vi "UI.vi"(0 "reference in":refnum<class "GUI OIL_FILLING.lvclass">, 5 "error in (no error)":errorcluster) -> (14 "reference out":refnum<class "GUI OIL_FILLING.lvclass">, 19 "error out":errorcluster)   [LabVIEW 2019, in "GUI OIL_FILLING.lvclass"]
uses:
  GUI OIL_FILLING.lvclass
  D:/H4000/src/GUI_class/GUI.lvclass
  GUI_class/GUI.lvclass/GUI.ctl
  TypeDef/AI_Data_Array.ctl
  TypeDef/AI_Data.ctl
  SV_Wrap/SharedVariableWrapper.lvclass/SharedVariableWrapper.ctl
  TypeDef/State.ctl
  MessageAMC_class/MessageAMC.lvclass
  D:/H4000/src/MessageInterface_class/MessageInterface.lvclass
  60afc6ad-d234-470a-b2ea-5a97dad0136d.vi
  94cfafae-4fb1-41fa-8c91-5db137de6dca.vi
  1b4fed76-272f-4eb9-b435-1b7916789d73.vi
  d0ca9bf2-7cd9-4c29-a03d-de1c10393a74.vi
  GUI_class/Set Win State.vi
  94cfafae-4fb1-41fa-8c91-5db137de6dca.vi/4db0cfde-7309-4fb5-ba82-78d4deda94bf.vi
  SV_Wrap/Write Var Info.vi
  SV_Wrap/Read Var Info.vi
  1b4fed76-272f-4eb9-b435-1b7916789d73.vi/fad6aa2d-1fd6-40e9-9208-cebdd25b163b.vi
  d0ca9bf2-7cd9-4c29-a03d-de1c10393a74.vi/ea186c4c-0445-4979-bfc0-5907181f2b8f.vi
  SV_Wrap/Read connection str.vi
  <userlib>/_OpenG.lib/time/time.llb/Tick Count (ms)__ogtk.vi
  TypeDef/GUI Setting Channel.ctl
  GUI_class/GUI.lvclass
  ConfigInterface_class/ConfigInterface.lvclass
  d678bd6a-011c-496f-8712-f7d087665a22.vi
  8e32a023-0563-484b-b85f-c3305c0d5712.vi
  MessageInterface_class/MessageInterface.lvclass
  SV_Wrap/SharedVariableWrapper.lvclass
panel:
  out "State":string
  in  "Set SP":bool
  in  "Setpoint":dbl caption="Давление прокачки"
  in  "Stop Button":bool
  in  "Start Button":bool
  out "AI 9":dbl(knob) caption="Давление  в  линии подачи \nвоздуха после БПВ" scale=0.0..16.0
  out "AI 8":dbl(knob) caption="Давление  в  линии подачи \nвоздуха в БПВ" scale=0.0..16.0
  out "DI 11":bool caption="БП [G2]"
  out "DI 8":bool caption="QF9"
  out "DI 7":bool caption="QF8"
  out "DI 6":bool caption="QF7"
  out "DI 5":bool caption="QF6"
  out "DI 4":bool caption="QF5"
  out "DI 3":bool caption="QF4"
  out "DI 2":bool caption="QF3"
  out "DI 1":bool caption="QF2"
  out "DI 0":bool caption="QF1"
  out "Connect":bool
  in  "Reset Alarms":bool
  in  "stop":bool
  out "DI 10":bool caption="БП [G1]"
  out "DI 9":bool caption="РКФ"
  # "Автоматы"
  # "0 - не готов\n1 -готов к запуска\n2 - пуск\n3 -качает\n4 - отскановка"
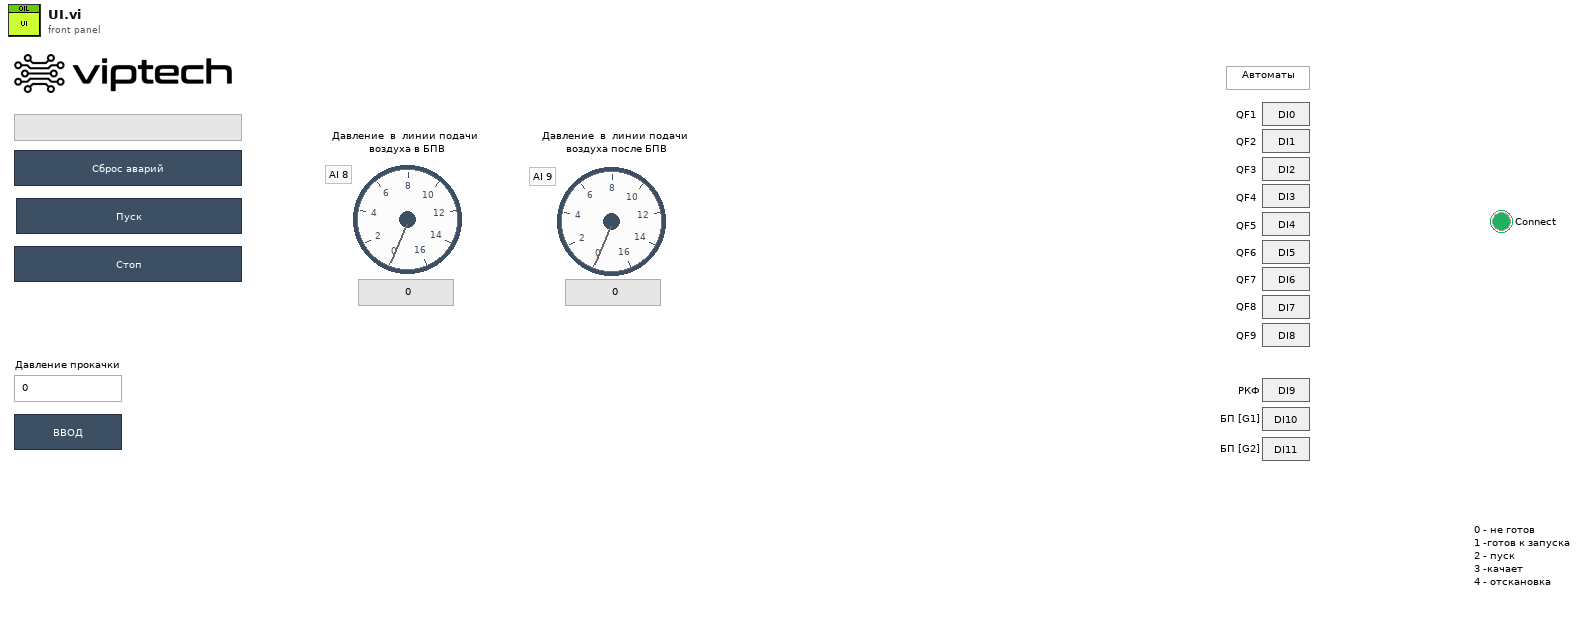
[diagram p1: front panel]
types:
  T1 = typedef "State.ctl" = enum16{"INIT", "IDLE", "CHANNEL_TESTING", "OIL_FILLING", "PREPARE_TO_HI_PRESS", "HI_PRESSURE", "ALARM", "HI PRESSURE TEST"}
  T2 = enum32{"Invalid", "Standard", "Closed", "Hidden", "Minimized", "Maximized"}
  T3 = enum32{"invalid app kind", "Development System", "Run Time System", "Student Edition", "Embedded LabVIEW", "Evaluation", "Custom"}
  T4 = typedef "GUI Setting Channel.ctl" = cluster{"Name":string, "SensorID":u32}
  T5 = typedef "GUI.lvclass/Shered Data.ctl" = cluster{"WindowsState":T6, "UI VI":refnum<vi>, "SubPnl":refnum<vi>}
  T6 = typedef "GUI.lvclass/WindowsState.ctl" = enum16{"NotReady", "Ready", "Inserted", "Opened"}
  T7 = typedef "SharedVariableWrapper.lvclass/Config.ctl" = cluster{"connection str":string, "timeout":dbl, "ip":string}
  T8 = cluster{"Core":cluster{"Current VI Reference":refnum<vi>, "Close Panel on Exit?":bool}, "amc":refnum<class "MessageAMC.lvclass">}
  T9 = cluster{"Current VI Reference":refnum<vi>, "Close Panel on Exit?":bool}
  T10 = typedef "GUI Alarm customer settings.ctl" = cluster{"HIHI AI2":dbl, "HI AI2":dbl, "HIHI AI3":dbl, "HI AI3":dbl, "ENG0 OFF TIMEOUT":dbl, "ENG0 ON TIMEOUT":dbl, "HIHI AI7":dbl, "HI AI7":dbl, "HIHI AI6":dbl, "HI AI6":dbl, "HIHI AI5":dbl, "HI AI5":dbl}
  T11 = typedef "GUI Alarm developer settings.ctl" = cluster{"HIHI AI2":dbl, "HI AI2":dbl, "HIHI AI0":dbl, "HI AI0":dbl, "LOLO AI0":dbl, "LO AI0":dbl, "ENG2 OFF TIMEOUT":dbl, "ENG2 ON TIMEOUT":dbl, "HIHI AI3":dbl, "HI AI3":dbl, "HIHI AI1":dbl, "HI AI1":dbl, "LOLO AI1":dbl, "LO AI1":dbl, "ENG1 OFF TIMEOUT":dbl, "ENG1 ON TIMEOUT":dbl, "ENG0 OFF TIMEOUT":dbl, "ENG0 ON TIMEOUT":dbl, "LOLO AI8":dbl, "LO AI8":dbl, "LOLO AI9":dbl, "LO AI9":dbl, "LOLO AI5":dbl, "LO AI5":dbl, "Out Of Range HI":dbl, "Out Of Range LO":dbl}
  T12 = typedef "AI_Data_Array.ctl" = T13[]
  T13 = typedef "AI_Data.ctl" = cluster{"Raw":dbl, "Scaled":dbl, "OutOfRangeMax":bool, "OutOfRangeMin":bool, "HIHI":bool, "HI":bool, "LO":bool, "LOLO":bool, "OutOfRangeMax_val":dbl, "OutOfRangeMin_val":dbl, "HIHI_val":dbl, "HI_val":dbl, "LO_val":dbl, "LOLO_val":dbl}
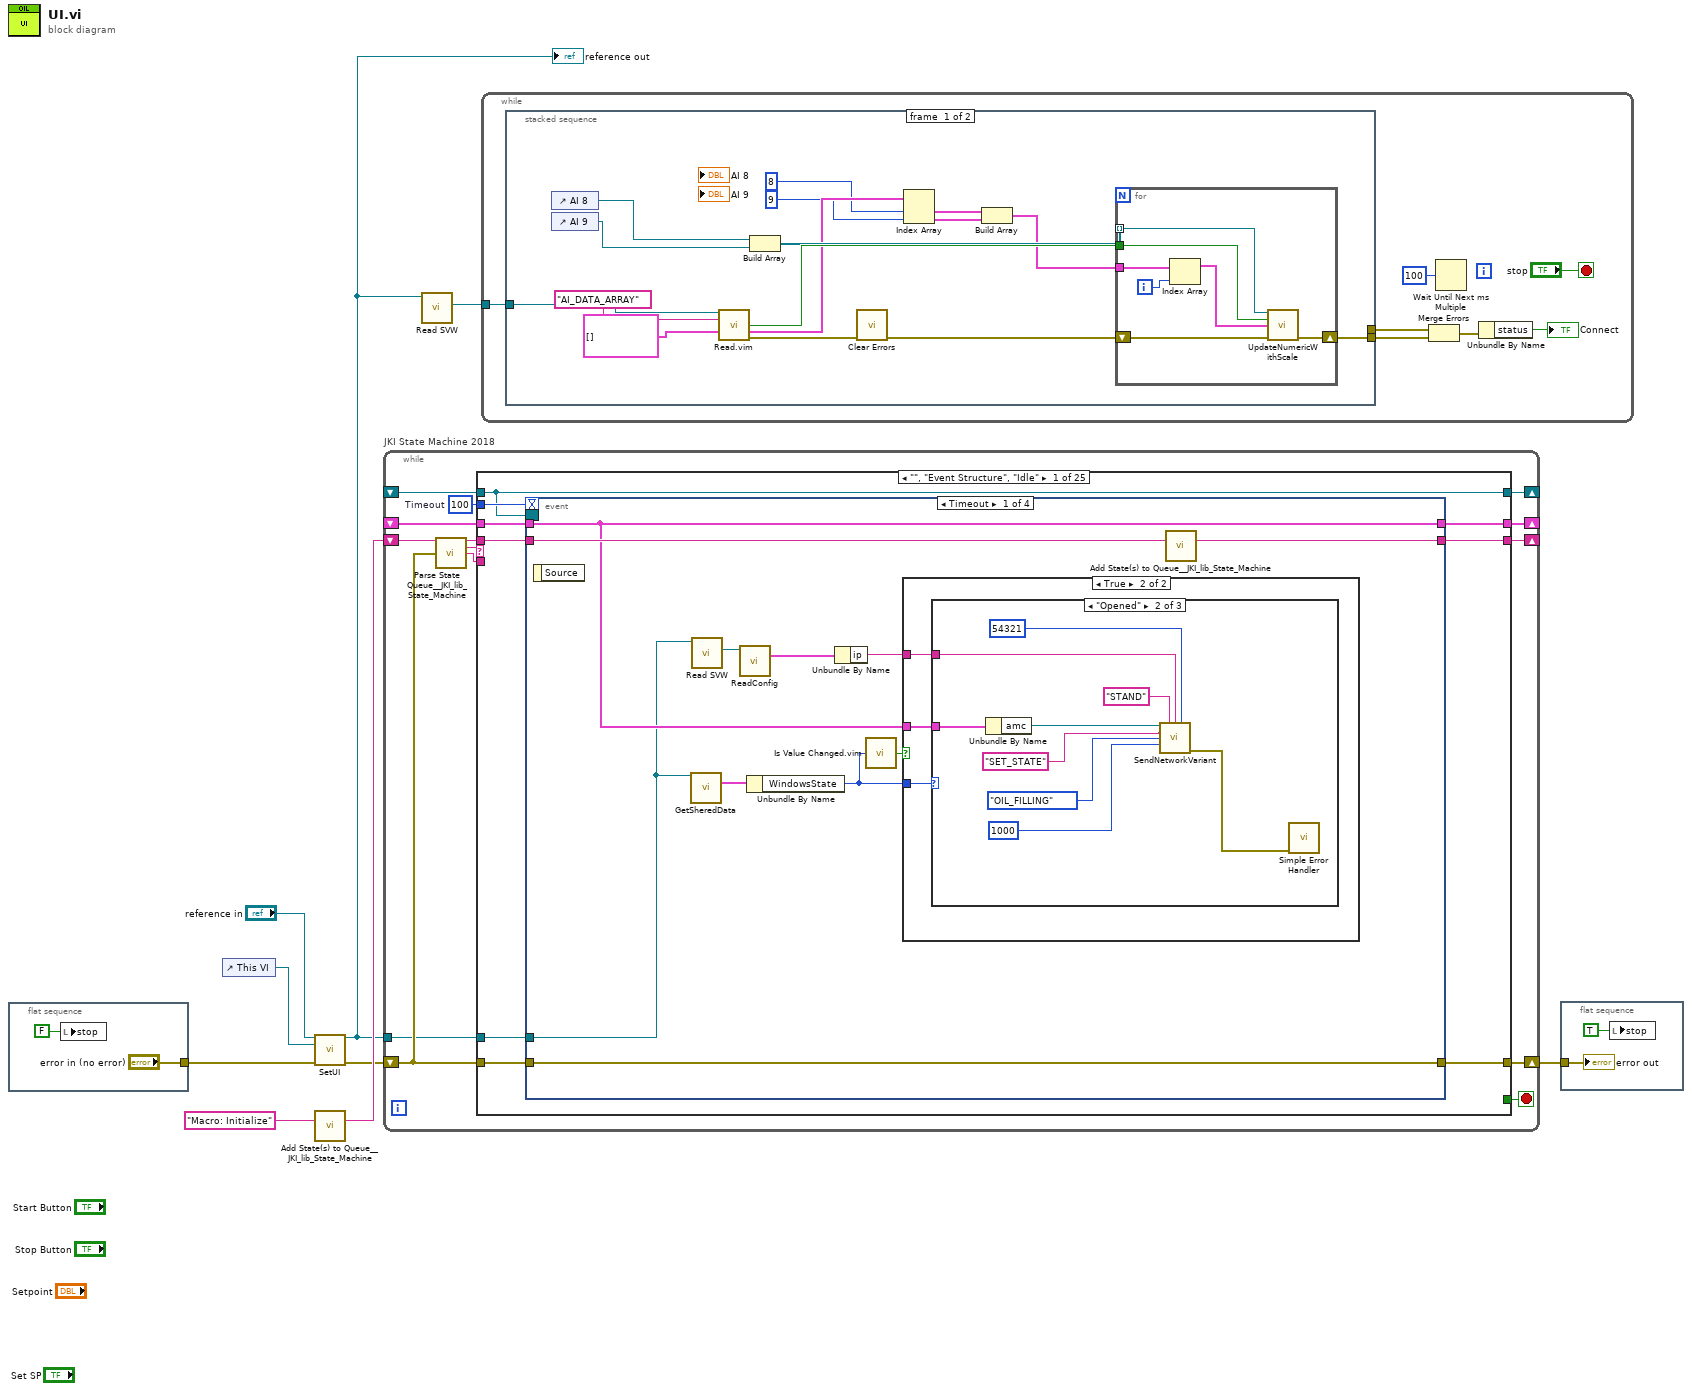
[diagram p0: block diagram]
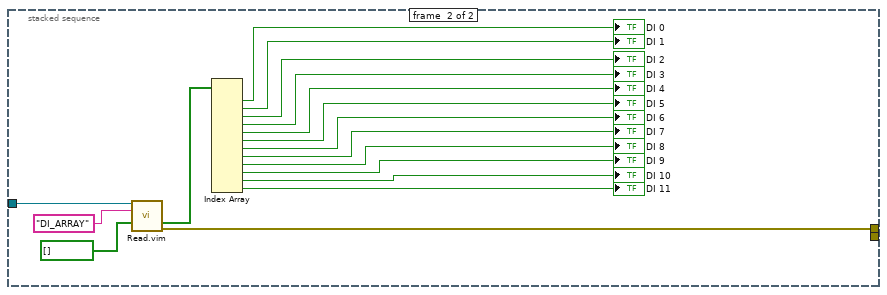
[diagram p2: hidden frame]
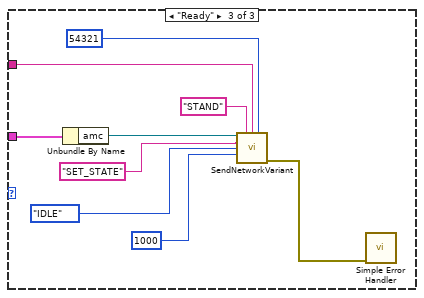
[diagram p5: hidden frame]
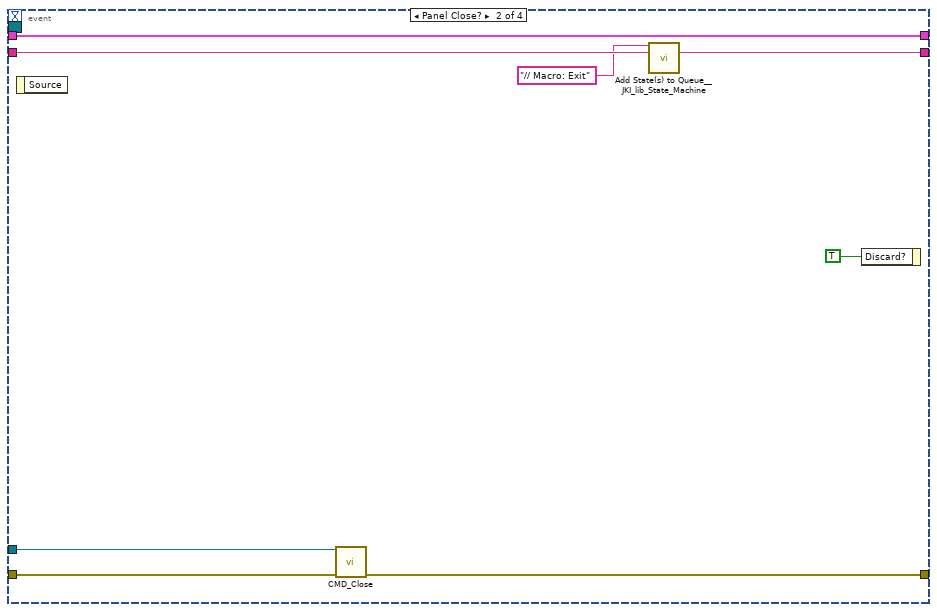
[diagram p6: hidden frame]
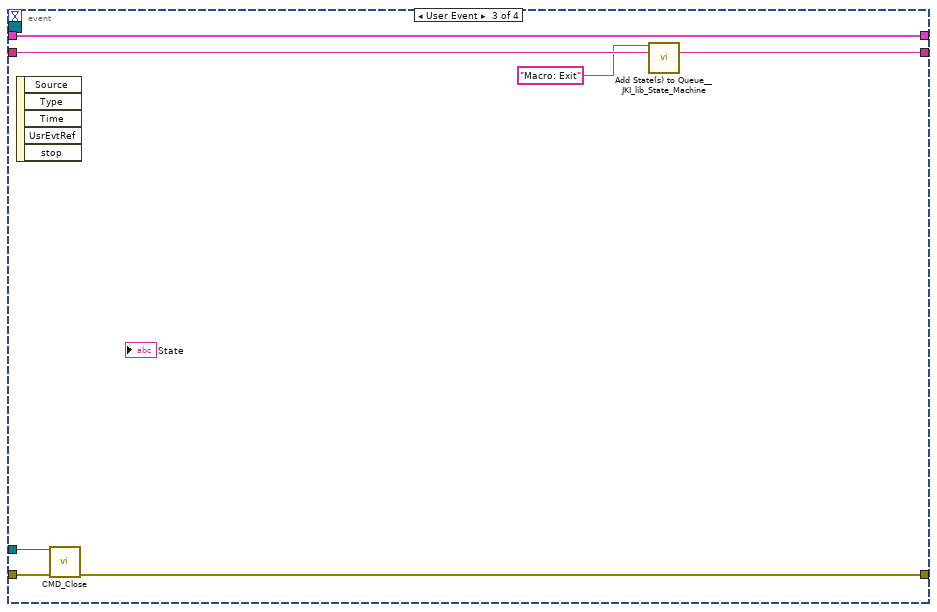
[diagram p7: hidden frame]
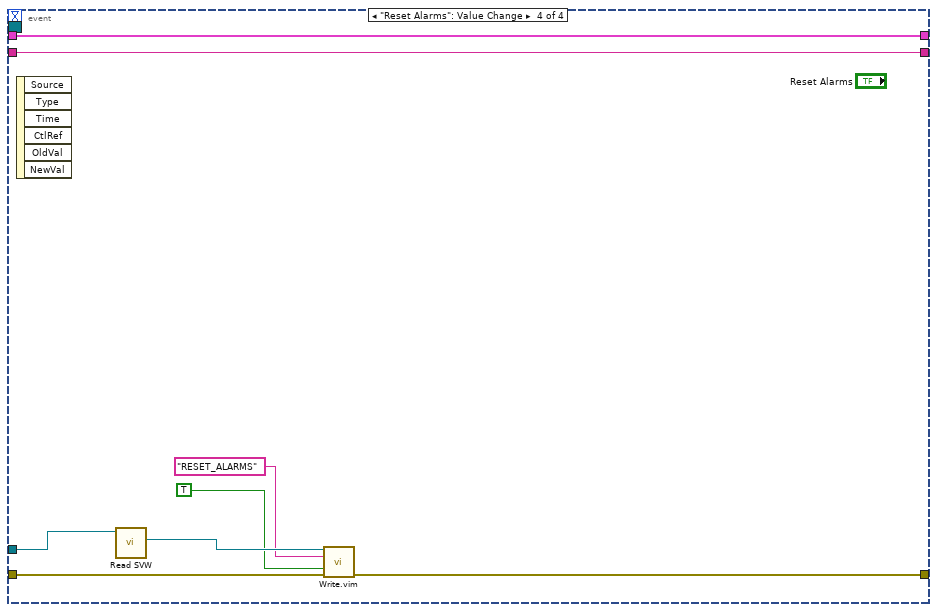
[diagram p8: hidden frame]
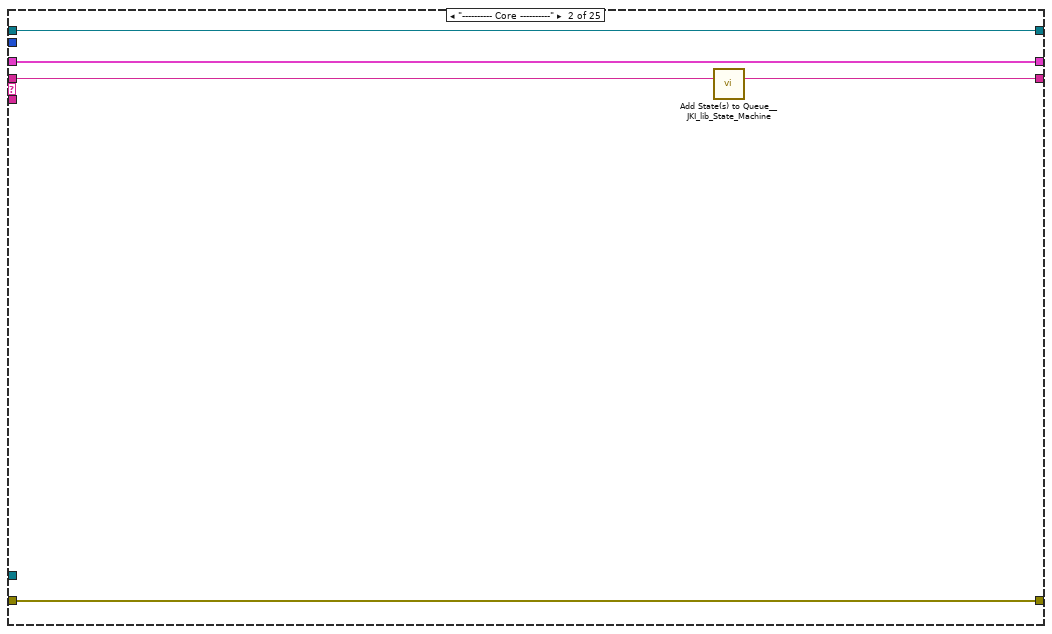
[diagram p9: hidden frame]
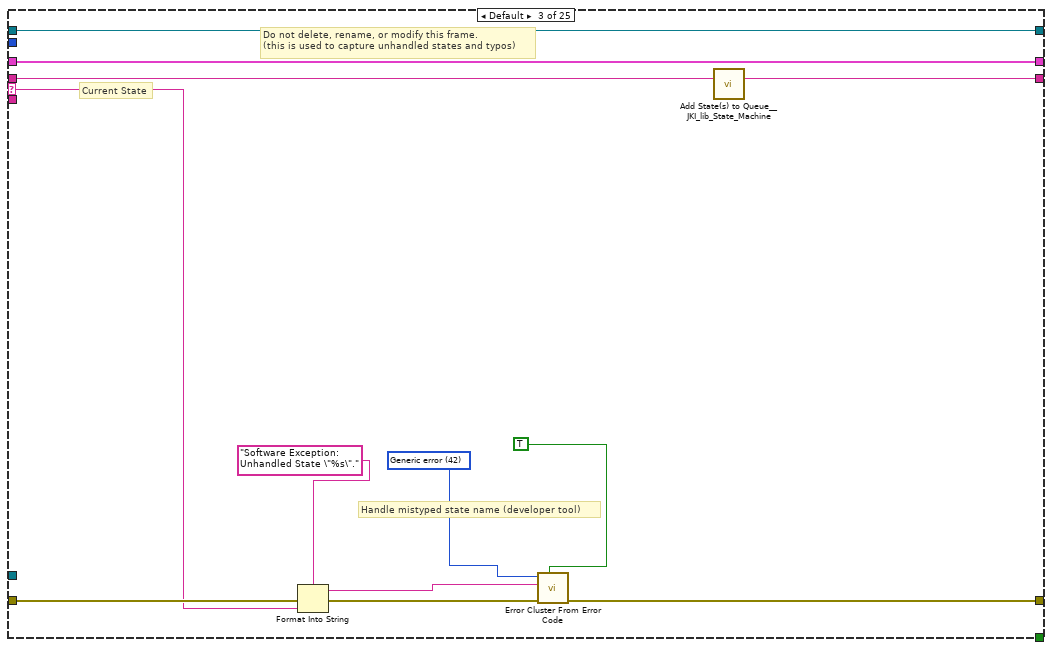
[diagram p10: hidden frame]
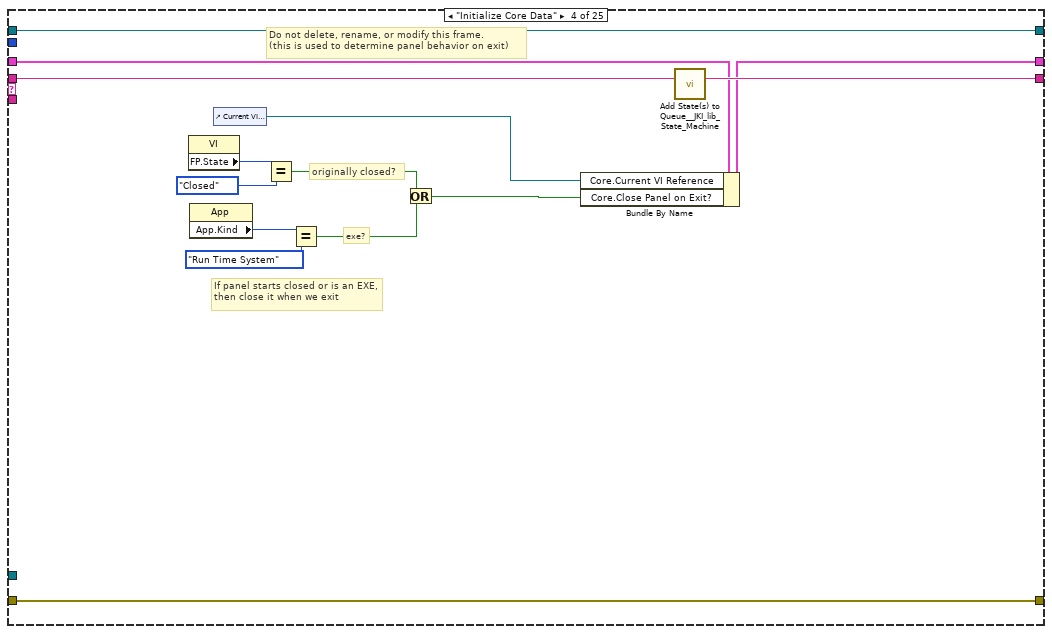
[diagram p11: hidden frame]
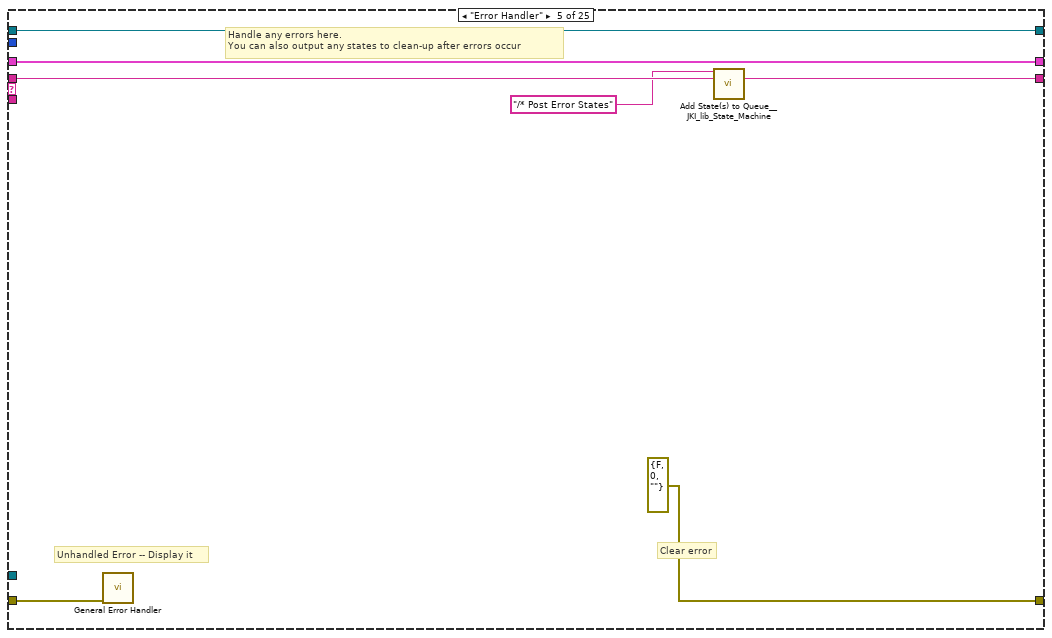
[diagram p12: hidden frame]
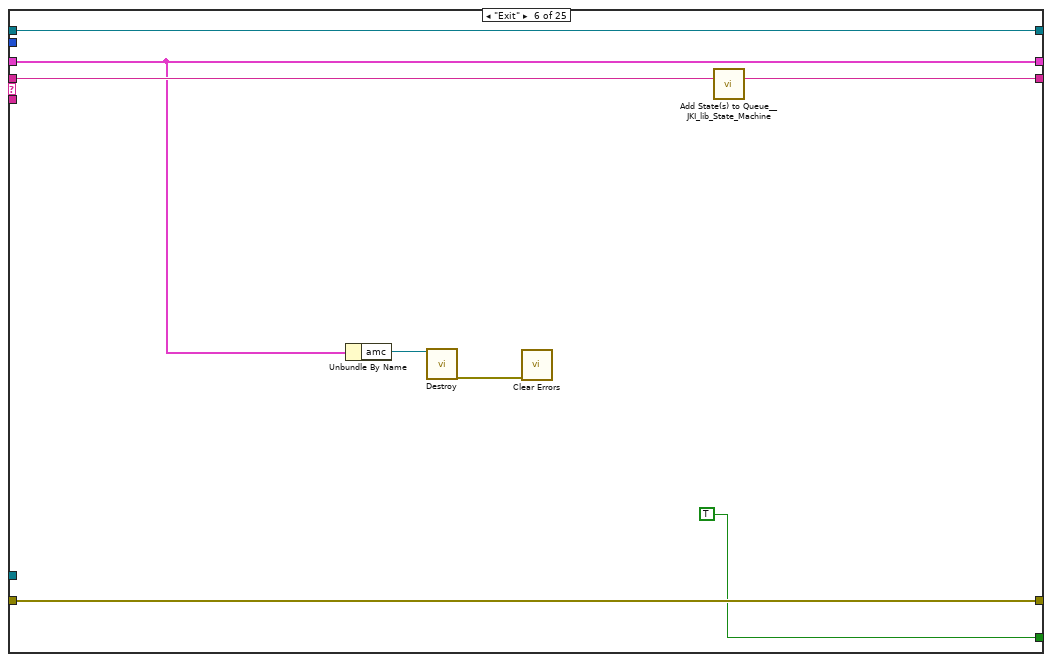
[diagram p13: hidden frame]
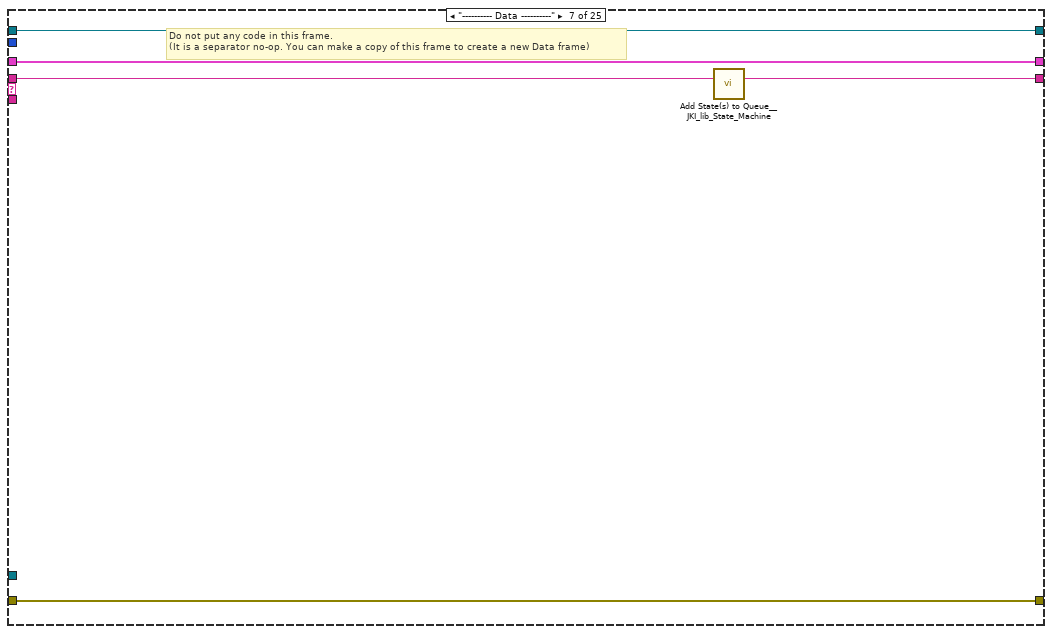
[diagram p14: hidden frame]
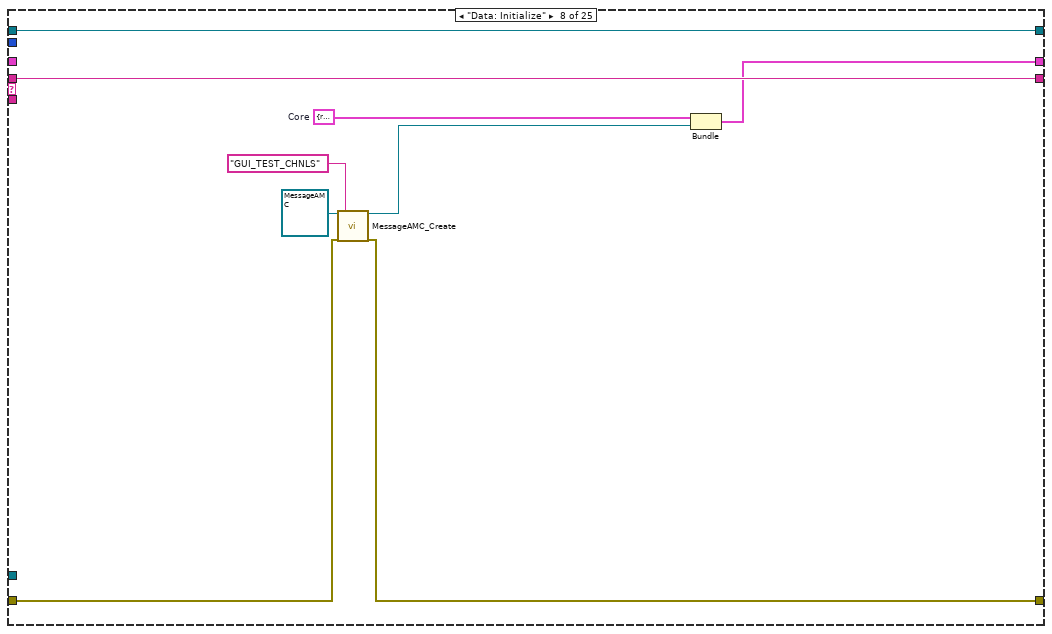
[diagram p15: hidden frame]
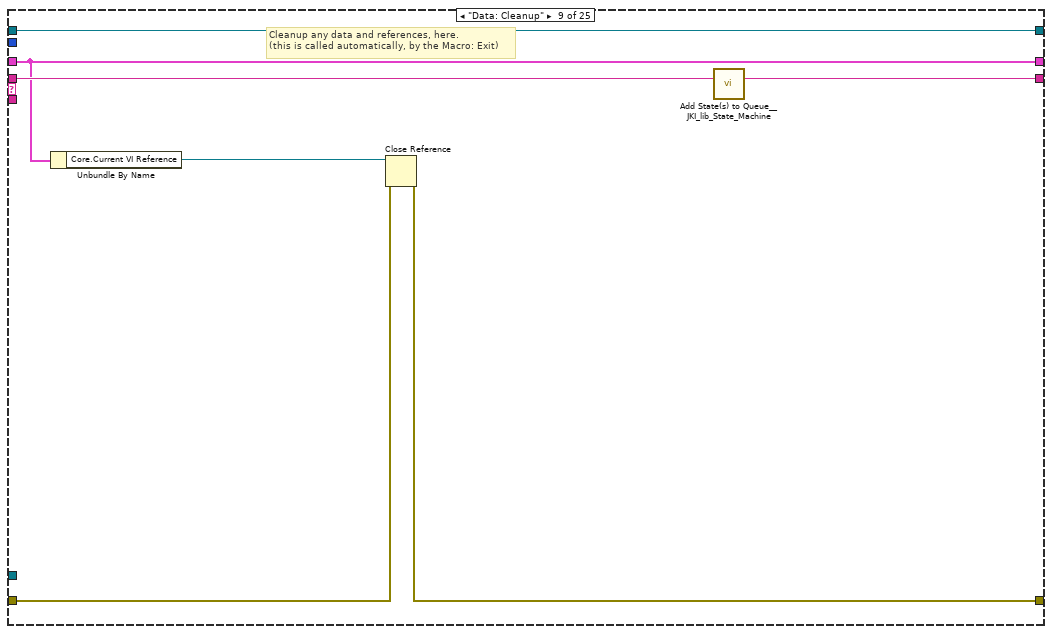
[diagram p16: hidden frame]
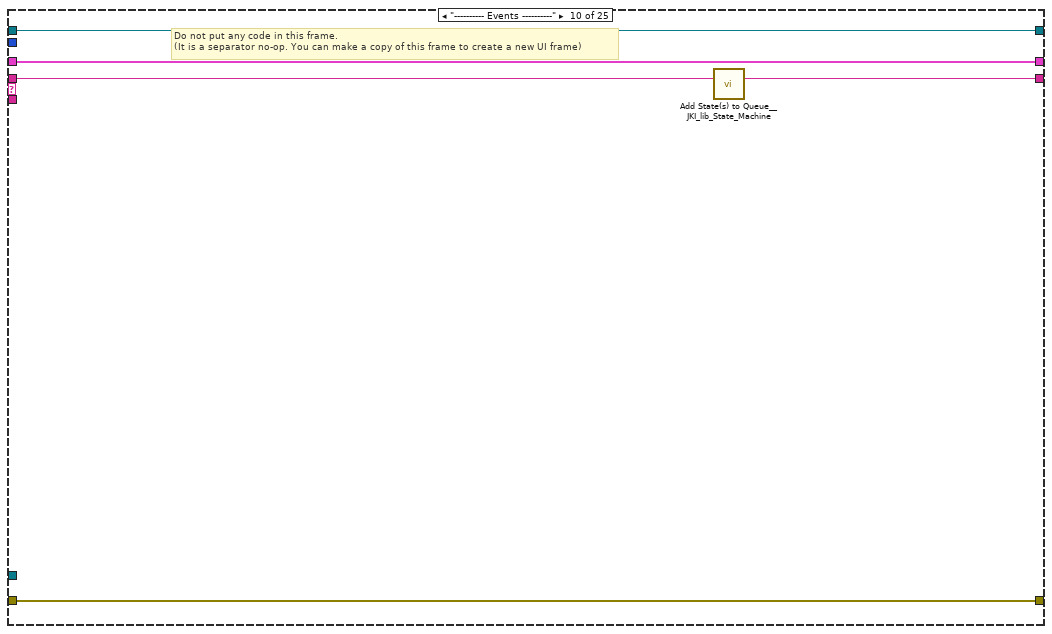
[diagram p17: hidden frame]
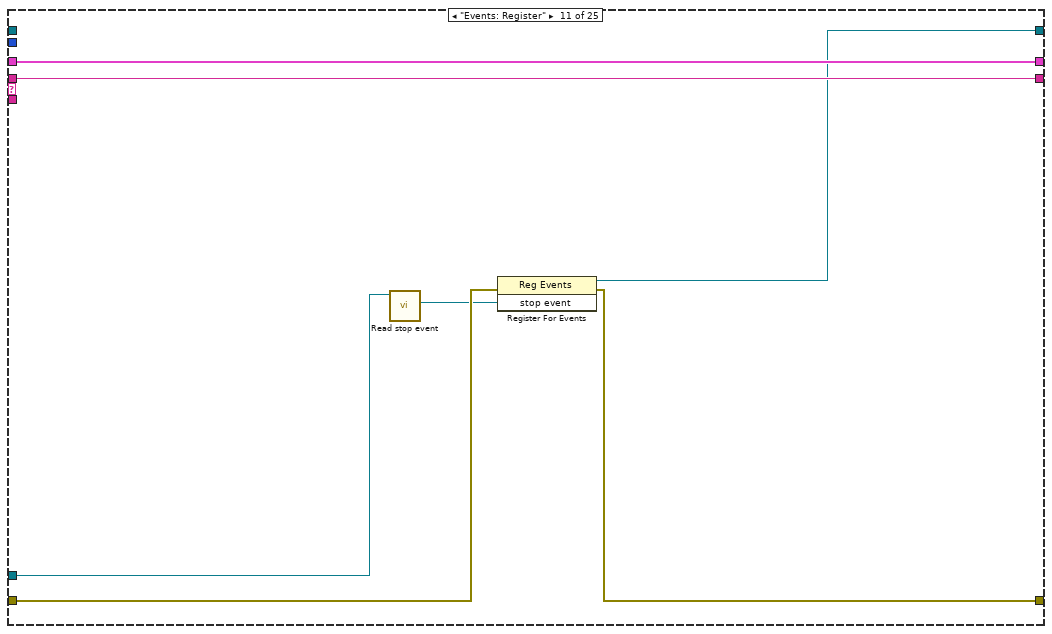
[diagram p18: hidden frame]
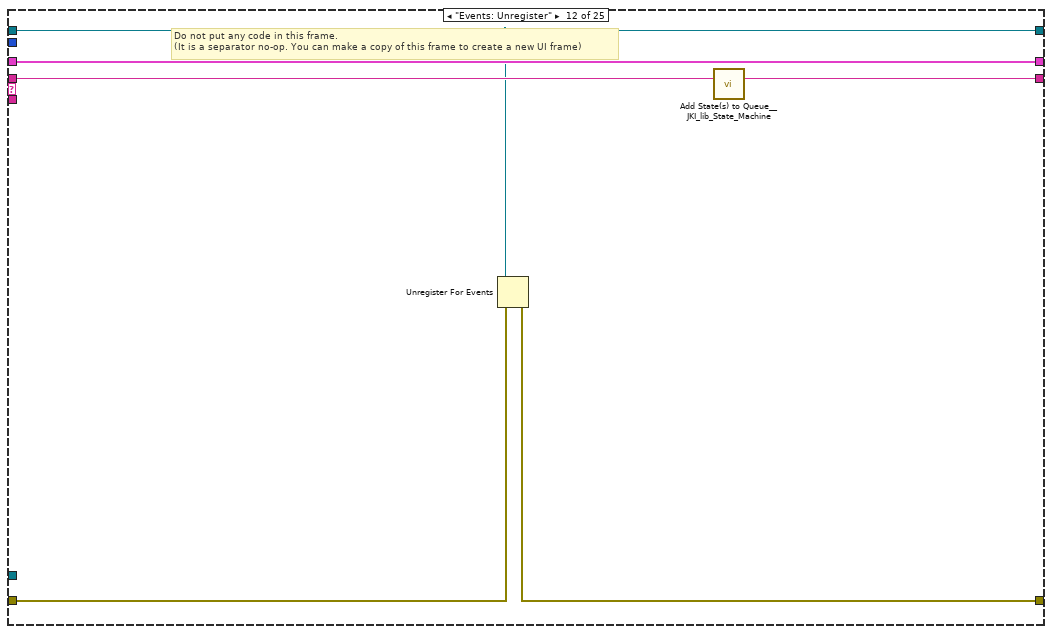
[diagram p19: hidden frame]
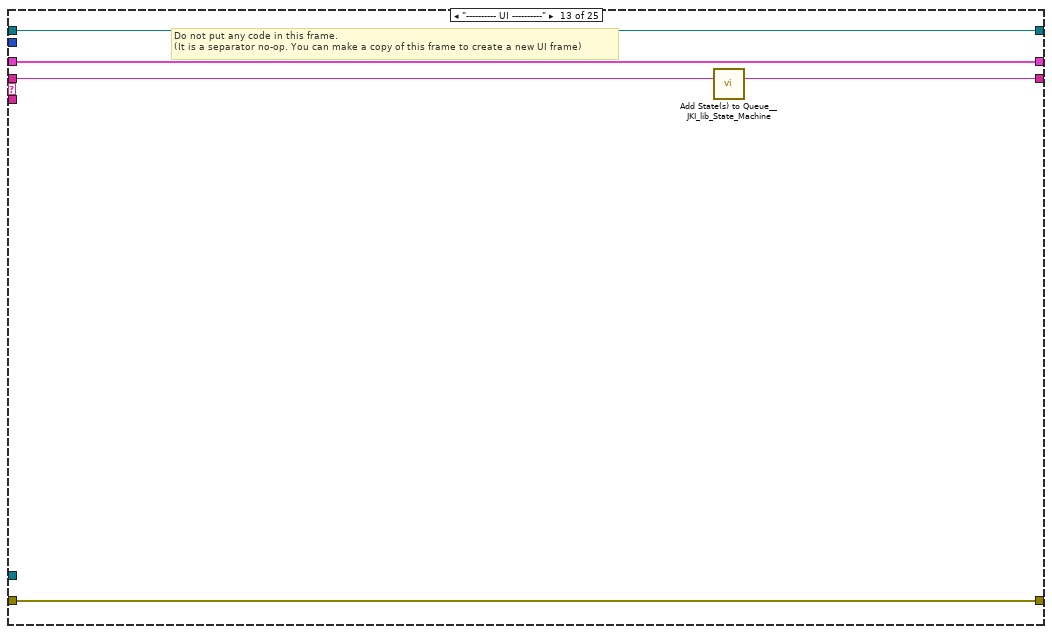
[diagram p20: hidden frame]
diagram:
  n1 = flat-sequence {
    tunnel: ["error in (no error)"] -> w6
    frame #0 {
      n2 = local write "stop"(FALSE ("stop")) -> ()
    }
  }
  n3 = control-ref of="This VI"() -> (w4:refnum<vi>)
  n4 = call "SetUI.vi"("reference in"="reference in", "UI VI"=w4, "error in (no error)"=w6) -> ("reference out"=w2:refnum<class "GUI OIL_FILLING.lvclass">, "error out"=w3:errorcluster)  [unwired: 11 in]
  "reference out" <- w2
  n5 = call <vilib>:"Add State(s) to Queue__JKI_lib_State_Machine.vi"("State(s) in (\"\")"="Macro: Initialize") -> ("States Out"=w9:string)  [unwired: 14 in]
  n6 = while "JKI State Machine 2018" {
    shift-right: [w18] -> _
    shift-left: _ -> [w17]
    shift-right: [w21] -> w7
    shift-left: w3 -> [w15]
    shift-right: [w20] -> _
    shift-left: w9 -> [w22]
    tunnel: w2 -> [w14]
    shift-right: [w13] -> _
    shift-left: _ -> [w12]
    stop <- w19 stop-if-true
    w16 = 100  # Timeout
    n7 = call <vilib>:"Parse State Queue__JKI_lib_State_Machine.vi"("State Queue"=w22, "Error In (no error)"=w15) -> ("Remaining States"=w24:string, "Current State"=w25:string, "Arguments"=w23:string)  [unwired: 11 in]
    n8 = case shown="\"\", \"Event Structure\", \"Idle\"" w25 {
      selector: w25 -> [_ _ w96 _ _ _ _ _ _ _ _ _ _ _ _ _ _ _ _ _ _ _ _ _ _]
      tunnel: w24 -> [w34 w94 w100 w120 w127 w135 w140 w149 w156 w161 w168 w174 w179 w183 w190 w202 w272 w278 w284 w296 w300 w301 w333 w349 w351]
      tunnel: w23 -> [_ _ _ _ _ _ _ _ _ _ _ _ _ _ w185 w196 _ _ _ _ _ _ _ _ _]
      tunnel: w17 -> [w32 w91 w98 w113 w124 w130 w137 _ w151 w158 w167 w172 w176 w182 w188 w198 w269 w275 w281 w293 w298 w304 w329 w346 w350]
      tunnel: [w31 w92 w102 w117 errorcluster {"status"=FALSE, "code"=0, "source"=""} ("error out") w133 w138 w142 w152 w159 w165 w169 w177 w181 w186 w199 w270 w276 w282 w294 w299 w305 w328 w347 w353] -> w21
      tunnel: w15 -> [w30 w92 w101 w117 w123 w133 w138 w143 w153 w159 w164 w170 w177 w181 w187 w200 w270 w276 w282 w294 w299 w306 w330 w347 w353]
      tunnel: [w33 w93 w99 w119 w126 w134 w139 w149 w155 w160 w168 w173 w178 w183 w189 w201 w271 w277 w283 w295 w300 w302 w333 w349 w351] -> w20
      tunnel: [_ _ _ _ _ TRUE _ _ _ _ _ _ _ _ _ _ _ _ _ _ _ _ _ _ _] -> w19
      tunnel: [w29 w91 w98 w118 w124 w130 w137 w148 w151 w158 w167 w172 w176 w182 w188 w198 w269 w275 w281 w293 w298 w303 w329 w346 w350] -> w18
      tunnel: w16 -> [w28 _ _ _ _ _ _ _ _ _ _ _ _ _ _ _ _ _ _ _ _ _ _ _ _]
      tunnel: w14 -> [w27 _ _ _ _ _ _ _ _ _ w163 _ _ _ _ _ _ _ _ _ _ w308 w331 _ _]
      tunnel: [w26 w90 w95 w107 w121 w131 w136 w146 w150 w157 w166 w171 w175 w180 w184 w195 w268 w273 w279 w286 w297 w309 w332 w348 w352] -> w13
      tunnel: w12 -> [w26 w90 w95 w107 w121 w131 w136 w146 w150 w157 _ w171 w175 w180 w184 w195 w268 w273 w279 w286 w297 w309 w332 w348 w352]
      frame "", "Event Structure", "Idle" {
        n9 = event shown="[0] Timeout" {
          selector: w26 -> [_ _ _ _]
          dyn-events: _ -> [_ _ _ _]
          timeout: w28 -> [_ _ _ _]
          tunnel: w34 -> [w45 w74 w81 w89]
          tunnel: [w44 w73 w80 w89] -> w33
          tunnel: w32 -> [w39 w72 w79 w88]
          tunnel: [w43 w67 w75 w82] -> w31
          tunnel: w30 -> [w43 w68 w76 w83]
          tunnel: [w39 w72 w79 w88] -> w29
          tunnel: w27 -> [w38 w69 w77 w87]
          event Timeout {
            n10 = event-data() -> ()  [unwired: 1 in, 1 out]
            n11 = call "GetSheredData.vi"("reference in"=w38) -> ("data"=w37:T5)  [unwired: 12 in, 2 out]
            n12 = call "Read SVW.vi"("GUI in"=w38) -> ("SharedVariableWrapper.lvclass"=w42:refnum<class "SharedVariableWrapper.lvclass">)  [unwired: 10 in]
            n13 = call "ReadConfig.vi"("SharedVariableWrapper in"=w42) -> ("config"=w41:T7)  [unwired: 12 in, 2 out]
            n14 = Unbundle By Name(w37) -> ("WindowsState"=w36:T6)
            n15 = Unbundle By Name(w41) -> ("ip"=w40:string)
            n16 = call "Is Value Changed.vim"("value"=w36) -> ("changed or first call?"=w35:bool)
            n17 = case shown="True" w35 {
              tunnel: w40 -> [_ w48]
              tunnel: w39 -> [_ w47]
              tunnel: w36 -> [_ w46]
              frame False {
              }
              frame True {
                n18 = case shown="\"Opened\"" w46 {
                  tunnel: w47 -> [_ w57 w66]
                  tunnel: w48 -> [_ w50 w59]
                  frame Default {
                  }
                  frame "Opened" {
                    n19 = Unbundle By Name(w57) -> ("amc"=w56:refnum<class "MessageAMC.lvclass">)
                    n20 = call "SendNetworkVariant.vi"("reference in"=w56, "receiver process"="STAND", "receiver host"=w50, "receiver port (0)"=u16 54321, "name"="SET_STATE", "data"=State."OIL_FILLING" ("State"), "timeout (25000 ms)"=1000) -> ("error out"=w52:errorcluster)  [unwired: 6 in, 2 out]
                    n21 = call <vilib>:"Simple Error Handler.vi"("error in (no error)"=w52) -> ()  [unwired: 4 in, 5 out]
                  }
                  frame "Ready" {
                    n22 = Unbundle By Name(w66) -> ("amc"=w65:refnum<class "MessageAMC.lvclass">)
                    n23 = call "SendNetworkVariant.vi"("reference in"=w65, "receiver process"="STAND", "receiver host"=w59, "receiver port (0)"=u16 54321, "name"="SET_STATE", "data"=State."IDLE" ("State"), "timeout (25000 ms)"=1000) -> ("error out"=w61:errorcluster)  [unwired: 6 in, 2 out]
                    n24 = call <vilib>:"Simple Error Handler.vi"("error in (no error)"=w61) -> ()  [unwired: 4 in, 5 out]
                  }
                }
              }
            }
            n25 = call <vilib>:"Add State(s) to Queue__JKI_lib_State_Machine.vi"("State(s) in (\"\")"=w45) -> ("States Out"=w44:string)  [unwired: 14 in]
          }
          event Panel Close? {
            n26 = event-data() -> ()  [unwired: 1 in, 1 out]
            n27 = call "CMD_Close.vi"("reference in"=w69, "error in (no error)"=w68) -> ("error out"=w67:errorcluster)  [unwired: 12 in, 1 out]
            n28 = call <vilib>:"Add State(s) to Queue__JKI_lib_State_Machine.vi"("State(s) in Front (\"\")"="// Macro: Exit", "State(s) in (\"\")"=w74) -> ("States Out"=w73:string)  [unwired: 13 in]
            n29 = event-data("Discard?"=TRUE) -> ()  [unwired: 1 in, 1 out]
          }
          event User Event {
            n30 = event-data() -> ()  [unwired: 1 in, 5 out]
            n31 = call "CMD_Close.vi"("reference in"=w77, "error in (no error)"=w76) -> ("error out"=w75:errorcluster)  [unwired: 12 in, 1 out]
            n32 = call <vilib>:"Add State(s) to Queue__JKI_lib_State_Machine.vi"("State(s) in Front (\"\")"="Macro: Exit", "State(s) in (\"\")"=w81) -> ("States Out"=w80:string)  [unwired: 13 in]
          }
          event "Reset Alarms": Value Change {
            n33 = event-data() -> ()  [unwired: 1 in, 6 out]
            n34 = call "Read SVW.vi"("GUI in"=w87) -> ("SharedVariableWrapper.lvclass"=w86:refnum<class "SharedVariableWrapper.lvclass">)  [unwired: 10 in]
            n35 = call "Write.vim"("SharedVariableWrapper in"=w86, "name"="RESET_ALARMS", "Data"=TRUE, "error in (no error)"=w83) -> ("error out"=w82:errorcluster)  [unwired: 5 in, 6 out]
          }
        }
      }
      frame "---------- Core ----------" {
        n36 = call <vilib>:"Add State(s) to Queue__JKI_lib_State_Machine.vi"("State(s) in (\"\")"=w94) -> ("States Out"=w93:string)  [unwired: 14 in]
      }
      frame Default {
        w105 = 42 items=["No error", "Argument error", "Memory is full", "Out of zone", "End of file", "File already open", "Generic file I/O error", "File not found", "File permission error", "Disk is full", "Duplicate path", "Too many files open", "System feature not enabled", "Resource file not found", "Cannot add resource", "Resource not found", "Image not found", "Image memory error", "Pen does not exist", "Config type invalid", "Config token not found", "Config parse error", "Config memory error", "Bad external code format", "Bad external code offset", "External code not present", "Null window", "Destroy window error", "Null menu", "Print aborted", "Bad print record", "Print driver error", "Windows error during printing", "Memory error during printing", "Print dialog error", "Generic print error", "Invalid device refnum", "Device not found", "Device parameter error", "Device unit error", "Cannot open device", "Device call aborted", "Generic error", "Cancelled by user", "Object ID too low", "Object ID too high", "Object not in heap", "Unknown heap", "Unknown object (invalid DefProc)", "Unknown object (DefProc not in table)", "Message out of range", "Invalid (null) method", "Unknown message", "Manager call not supported", "Bad address", "Network operation in progress", "Network operation timed out", "Connection is busy", "Network attribute not supported", "Network error", "Address in use", "System out of memory", "Connection aborted", "Connection refused", "Not connected", "Already connected", "Connection closed", "Initialization error (interapplication manager)", "Bad occurrence", "Wait on unbound occurrence handler", "Occurrence queue overflow", "Datalog type conflict", "Unused", "Unrecognized type (interapplication manager)", "Memory corrupt", "Failed to make temporary DLL", "Old CIN version", "Drag socket not found", "Failed to load drop-object", "Failed to register OLE object", "Failed to release OLE object", "Format specifier type mismatch", "Unknown format specifier", "Too few format specifiers", "Too many format specifiers", "Scan failed", "Newer CIN version", "Error converting to variant", "Runtime menu error", "Password tampered", "Variant attribute not found", "Incompatible variant data type", "Event data is not available", "Event Store is not present", "Occurrence is not found", "Event Queue is not created", "Event info is not available", "Refnum passed is NULL", "Error retrieving Class GUID", "Error retrieving CoClass GUID", "Error retrieving TypeLib GUID.", "Bad built application magic bytes.", "Specific driver is different from the specific driver associated with the Logical Name.", "There is no session opened to the class driver.", "Max Error", "MAX - Error with config objects", "MAX - Error loading configuration", "MAX - Group not supported"]
        # "Current State"
        # "Do not delete, rename, or modify this frame.\n(this is used to capture unhandled states and typos)"
        # "Handle mistyped state name (developer tool)"
        n37 = Format Into String(format string="Software Exception: Unhandled State \"%s\"." ("message"), error in=w101, w96) -> (resulting string=w104:string, error out=w103:errorcluster)  [unwired: 1 in]
        n38 = call <vilib>:"Error Cluster From Error Code.vi"("show call chain? (False)"=TRUE, "error in (no error)"=w103, "error message (\"\")"=w104, "error code (0)"=w105) -> ("error out"=w102:errorcluster)  [unwired: 5 in]
        n39 = call <vilib>:"Add State(s) to Queue__JKI_lib_State_Machine.vi"("State(s) in (\"\")"=w100) -> ("States Out"=w99:string)  [unwired: 14 in]
      }
      frame "Initialize Core Data" {
        # "Do not delete, rename, or modify this frame.\n(this is used to determine panel behavior on exit)"
        # "originally closed?"
        # "exe?"
        # "If panel starts closed or is an EXE, then close it when we exit"
        n40 = property class="VI"() -> ("FP.State"=w110:T2)  [unwired: 2 in, 2 out]
        n41 = property class="App"() -> ("App.Kind"=w116:T3)  [unwired: 2 in, 2 out]
        n42 = control-ref of="Current VI Reference"() -> (w111:refnum<vi>)
        n43 = Equal?(x=w110, y=T2."Closed" ("Front Panel Window:State")) -> (x = y?=w108:bool)
        n44 = Equal?(x=w116, y=T3."Run Time System" ("Application:Kind")) -> (x = y?=w114:bool)
        n45 = Or(x=w108, y=w114) -> (x .or. y?=w112:bool)
        n46 = Bundle By Name(cluster=w113, "Core.Current VI Reference"=w111, "Core.Close Panel on Exit?"=w112) -> (w118:T8)
        n47 = call <vilib>:"Add State(s) to Queue__JKI_lib_State_Machine.vi"("State(s) in (\"\")"=w120) -> ("States Out"=w119:string)  [unwired: 14 in]
      }
      frame "Error Handler" {
        # "Unhandled Error -- Display it"
        # "Handle any errors here.\nYou can also output any states to clean-up after errors occur"
        # "Clear error"
        n48 = call <vilib>:"General Error Handler.vi"("error in (no error)"=w123) -> ()  [unwired: 10 in, 5 out]
        n49 = call <vilib>:"Add State(s) to Queue__JKI_lib_State_Machine.vi"("State(s) in Front (\"\")"="/* Post Error States", "State(s) in (\"\")"=w127) -> ("States Out"=w126:string)  [unwired: 13 in]
      }
      frame "Exit" {
        n50 = Unbundle By Name(w130) -> ("amc"=w129:refnum<class "MessageAMC.lvclass">)
        n51 = call-dynamic "Destroy.vi"("reference in"=w129) -> ("error out"=w128:errorcluster)  [unwired: 17 in, 1 out]
        n52 = call <vilib>:"Clear Errors.vi"("error in (no error)"=w128) -> ()  [unwired: 5 in, 2 out]
        n53 = call <vilib>:"Add State(s) to Queue__JKI_lib_State_Machine.vi"("State(s) in (\"\")"=w135) -> ("States Out"=w134:string)  [unwired: 14 in]
      }
      frame "---------- Data ----------" {
        # "Do not put any code in this frame.\n(It is a separator no-op. You can make a copy of this frame to create a new Data frame)"
        n54 = call <vilib>:"Add State(s) to Queue__JKI_lib_State_Machine.vi"("State(s) in (\"\")"=w140) -> ("States Out"=w139:string)  [unwired: 14 in]
      }
      frame "Data: Initialize" {
        w147 = T9 {"Current VI Reference"=refnum, "Close Panel on Exit?"=FALSE}  # Core
        n55 = call "MessageAMC_Create.vi"("reference in"=refnum<class "MessageAMC.lvclass"> refnum, "error in (no error)"=w143, "message queue name"="GUI_TEST_CHNLS") -> ("amc"=w144:refnum<class "MessageAMC.lvclass">, "error out"=w142:errorcluster)  [unwired: 15 in]
        n56 = Bundle("Core"=w147, "amc"=w144) -> (w148:T8)  [unwired: 1 in]
      }
      frame "Data: Cleanup" {
        # "Cleanup any data and references, here.\n(this is called automatically, by the Macro: Exit)"
        n57 = Unbundle By Name(w151) -> ("Core.Current VI Reference"=w154:refnum<vi>)
        n58 = Close Reference(reference=w154, error in (no error)=w153) -> (error out=w152:errorcluster)
        n59 = call <vilib>:"Add State(s) to Queue__JKI_lib_State_Machine.vi"("State(s) in (\"\")"=w156) -> ("States Out"=w155:string)  [unwired: 14 in]
      }
      frame "---------- Events ----------" {
        # "Do not put any code in this frame.\n(It is a separator no-op. You can make a copy of this frame to create a new UI frame)"
        n60 = call <vilib>:"Add State(s) to Queue__JKI_lib_State_Machine.vi"("State(s) in (\"\")"=w161) -> ("States Out"=w160:string)  [unwired: 14 in]
      }
      frame "Events: Register" {
        n61 = call "Read stop event.vi"("GUI in"=w163) -> ("stop event"=w162:refnum<user-event>)  [unwired: 8 in, 2 out]
        n62 = register-events(error in=w164, w162) -> (reference out=w166:refnum<event-registration>, error out=w165:errorcluster)  [unwired: 1 in]
      }
      frame "Events: Unregister" {
        # "Do not put any code in this frame.\n(It is a separator no-op. You can make a copy of this frame to create a new UI frame)"
        n63 = Unregister For Events(event registration refnum=w171, error in=w170) -> (error out=w169:errorcluster)
        n64 = call <vilib>:"Add State(s) to Queue__JKI_lib_State_Machine.vi"("State(s) in (\"\")"=w174) -> ("States Out"=w173:string)  [unwired: 14 in]
      }
      frame "---------- UI ----------" {
        # "Do not put any code in this frame.\n(It is a separator no-op. You can make a copy of this frame to create a new UI frame)"
        n65 = call <vilib>:"Add State(s) to Queue__JKI_lib_State_Machine.vi"("State(s) in (\"\")"=w179) -> ("States Out"=w178:string)  [unwired: 14 in]
      }
      frame "UI: Initialize" {
      }
      frame "UI: Cursor Set" {
        # "Argument"
        # "Set and Unset Cursor Busy.\n(Usage: \"UI: Cursor Set >> Busy|Idle\")"
        n66 = case shown="\"Idle\", Default" w185 {
          tunnel: w187 -> [w192 w194]
          tunnel: [w191 w193] -> w186
          frame "Idle", Default {
            n67 = call <vilib>:"Unset Busy.vi"("error in (no error)"=w192) -> ("error out"=w191:errorcluster)  [unwired: 10 in]
          }
          frame "Busy" {
            n68 = call <vilib>:"Set Busy.vi"("error in (no error)"=w194) -> ("error out"=w193:errorcluster)  [unwired: 9 in, 1 out]
          }
        }
        n69 = call <vilib>:"Add State(s) to Queue__JKI_lib_State_Machine.vi"("State(s) in (\"\")"=w190) -> ("States Out"=w189:string)  [unwired: 14 in]
      }
      frame "UI: Front Panel State" {
        # "Argument"
        # "Set Front Panel Open or Closed\n(Usage: \"UI: Front Panel State >> Open|Close\")"
        n70 = Unbundle By Name(w198) -> ("Core.Current VI Reference"=w197:refnum<vi>)
        n71 = case shown="\"Minimize\", \"Minimized\"" w196 {
          tunnel: w200 -> [w208 w223 w234 w247 w260]
          tunnel: [w210 w224 w236 w249 w262] -> w199
          tunnel: w197 -> [w209 w221 w235 w248 w261]
          frame "Open", "Standard", Default {
            w203 = T2."Standard" ("State")
            n72 = property class="VI"(reference=w209, error in=w208) -> (reference out=w206:refnum<vi>, error out=w207:errorcluster, "FP.State"=w205:T2)
            n73 = Not Equal?(x=w205, y=w203) -> (x != y?=w204:bool)
            n74 = case shown="True" w204 {
              tunnel: [w214 w216] -> w210
              tunnel: w207 -> [w213 w216]
              tunnel: w206 -> [w212 _]
              tunnel: w203 -> [w211 _]
              frame True {
                n75 = invoke class="VI" method="FP.Open"(reference=w212, error in=w213, "Activate"=TRUE, "State"=w211) -> (error out=w214:errorcluster)  [unwired: 1 in, 4 out]
              }
              frame False {
              }
            }
          }
          frame "Close", "Closed" {
            n76 = property class="VI"(reference=w221, error in=w223) -> (reference out=w220:refnum<vi>, error out=w222:errorcluster, "FP.State"=w218:T2)
            n77 = Not Equal?(x=w218, y=T2."Closed" ("Front Panel Window:State")) -> (x != y?=w217:bool)
            n78 = case shown="True" w217 {
              tunnel: [w225 w228] -> w224
              tunnel: w222 -> [w225 w227]
              tunnel: w220 -> [_ w226]
              frame False {
              }
              frame True {
                n79 = invoke class="VI" method="FP.Close"(reference=w226, error in=w227) -> (error out=w228:errorcluster)  [unwired: 1 in, 2 out]
              }
            }
          }
          frame "Hidden", "Hide" {
            w229 = T2."Hidden" ("State")
            n80 = property class="VI"(reference=w235, error in=w234) -> (reference out=w232:refnum<vi>, error out=w233:errorcluster, "FP.State"=w231:T2)
            n81 = Not Equal?(x=w231, y=w229) -> (x != y?=w230:bool)
            n82 = case shown="True" w230 {
              tunnel: [w240 w241] -> w236
              tunnel: w233 -> [w239 w241]
              tunnel: w232 -> [w238 _]
              tunnel: w229 -> [w237 _]
              frame True {
                n83 = invoke class="VI" method="FP.Open"(reference=w238, error in=w239, "State"=w237) -> (error out=w240:errorcluster)  [unwired: 2 in, 4 out]
              }
              frame False {
              }
            }
          }
          frame "Minimize", "Minimized" {
            w242 = T2."Minimized" ("State")
            n84 = property class="VI"(reference=w248, error in=w247) -> (reference out=w245:refnum<vi>, error out=w246:errorcluster, "FP.State"=w244:T2)
            n85 = Not Equal?(x=w244, y=w242) -> (x != y?=w243:bool)
            n86 = case shown="True" w243 {
              tunnel: [w253 w254] -> w249
              tunnel: w246 -> [w252 w254]
              tunnel: w245 -> [w251 _]
              tunnel: w242 -> [w250 _]
              frame True {
                n87 = invoke class="VI" method="FP.Open"(reference=w251, error in=w252, "State"=w250) -> (error out=w253:errorcluster)  [unwired: 2 in, 4 out]
              }
              frame False {
              }
            }
          }
          frame "Maximize", "Maximized" {
            w255 = T2."Maximized" ("State")
            n88 = property class="VI"(reference=w261, error in=w260) -> (reference out=w258:refnum<vi>, error out=w259:errorcluster, "FP.State"=w257:T2)
            n89 = Not Equal?(x=w257, y=w255) -> (x != y?=w256:bool)
            n90 = case shown="True" w256 {
              tunnel: [w266 w267] -> w262
              tunnel: w259 -> [w265 w267]
              tunnel: w258 -> [w264 _]
              tunnel: w255 -> [w263 _]
              frame True {
                n91 = invoke class="VI" method="FP.Open"(reference=w264, error in=w265, "State"=w263) -> (error out=w266:errorcluster)  [unwired: 2 in, 4 out]
              }
              frame False {
              }
            }
          }
        }
        n92 = call <vilib>:"Add State(s) to Queue__JKI_lib_State_Machine.vi"("State(s) in (\"\")"=w202) -> ("States Out"=w201:string)  [unwired: 14 in]
      }
      frame "---------- Macro ----------" {
        # "Do not put any code in this frame.\n(It is a separator no-op. You can make a copy of this frame to create a new Macro frame)"
        n93 = call <vilib>:"Add State(s) to Queue__JKI_lib_State_Machine.vi"("State(s) in (\"\")"=w272) -> ("States Out"=w271:string)  [unwired: 14 in]
      }
      frame "Macro: Initialize" {
        n94 = call <vilib>:"Add State(s) to Queue__JKI_lib_State_Machine.vi"("State(s) in Front (\"\")"="Data: Initialize\nInitialize Core Data\nEvents: Register\nUI: Initialize\n// UI: Front Panel State >> Open\n\n\nAction: Read Config\nAction: Update Indicators\n", "State(s) in (\"\")"=w278) -> ("States Out"=w277:string)  [unwired: 13 in]
      }
      frame "Macro: Update" {
        n95 = call <vilib>:"Add State(s) to Queue__JKI_lib_State_Machine.vi"("State(s) in Front (\"\")"="Action: Update Indicators\nAction: Write Config", "State(s) in (\"\")"=w284) -> ("States Out"=w283:string)  [unwired: 13 in]
      }
      frame "Macro: Exit" {
        # "Exit Macro\n(This is called once, when the VI exits)"
        n96 = Unbundle By Name(w293) -> ("Core.Close Panel on Exit?"=w292:bool)
        n97 = Select(t="UI: Front Panel State >> Close", s=w292, f="") -> (s? t:f=w289:string)
        n98 = call <vilib>:"Add State(s) to Queue__JKI_lib_State_Machine.vi"("State(s) in Front (\"\")"="Action: Write Config", "State(s) in (\"\")"=w289, "State(s) at Back (\"\")"="Data: Cleanup\nEvents: Unregister\nExit") -> ("States Out"=w287:string)  [unwired: 12 in]
        n99 = call <vilib>:"Add State(s) to Queue__JKI_lib_State_Machine.vi"("State(s) in Front (\"\")"=w287, "State(s) in (\"\")"=w296) -> ("States Out"=w295:string)  [unwired: 13 in]
      }
      frame "---------- Action ----------" {
      }
      frame "Action: Read Config" {
        n100 = call "Read ConfigInterface.vi"("GUI in"=w308) -> ("ConfigInterface"=w307:refnum<class "ConfigInterface.lvclass">)  [unwired: 9 in, 1 out]
        n101 = disable-structure shown="Enabled" {
          disable-tunnel: w307 -> [w314 _]
          disable-tunnel: w306 -> [w313 w326]
          disable-tunnel: [w312 w326] -> w305
          disable-tunnel: w304 -> [w311 w327]
          disable-tunnel: [w310 w327] -> w303
          frame Disabled {
            n102 = in-place {
              in-place-border: w314 -> [w325]
              in-place-border: w313 -> [w323]
              in-place-border: [w321] -> w312
              n103 = in-place-cluster #1(w311) -> ("GUI Alarm developer settings"=w318, "file developer"=w315, "GUI alarm customer settings"=w320, "file customer"=w316)
              n104 = call "ReadOrCreate.vim"("reference in"=w325, "Type and Defaults"=w320, "Name"=w316, "error in (no error)"=w323) -> ("reference out"=w324:refnum<class "ConfigInterface.lvclass">, "Data"=w319:T10, "error out"=w322:errorcluster)  [unwired: 7 in, 2 out]
              n105 = call "ReadOrCreate.vim"("reference in"=w324, "Type and Defaults"=w318, "Name"=w315, "error in (no error)"=w322) -> ("Data"=w317:T11, "error out"=w321:errorcluster)  [unwired: 7 in, 3 out]
              n106 = in-place-cluster #1("GUI Alarm developer settings"=w317, "file developer"=w315, "GUI alarm customer settings"=w319, "file customer"=w316) -> (w310:T8)
            }
          }
          frame Enabled {
          }
        }
        n107 = call <vilib>:"Add State(s) to Queue__JKI_lib_State_Machine.vi"("State(s) in (\"\")"=w301) -> ("States Out"=w302:string)  [unwired: 14 in]
      }
      frame "Action: Write Config" {
        n108 = disable-structure shown="Enabled" {
          disable-tunnel: w331 -> [w344 _]
          disable-tunnel: w330 -> [w342 w345]
          disable-tunnel: w329 -> [w341 _]
          disable-tunnel: [w336 w345] -> w328
          frame Disabled {
            n109 = Unbundle By Name(w341) -> ("GUI alarm customer settings"=w334, "file developer"=w335, "GUI Alarm developer settings"=w339, "file developer"=w340)
            n110 = call "Read ConfigInterface.vi"("GUI in"=w344) -> ("ConfigInterface"=w343:refnum<class "ConfigInterface.lvclass">)  [unwired: 9 in, 1 out]
            n111 = call-dynamic "Write.vi"("reference in"=w343, "Data"=w339, "Name"=w340, "error in (no error)"=w342) -> ("reference out"=w337:refnum<class "ConfigInterface.lvclass">, "error out"=w338:errorcluster)  [unwired: 8 in, 2 out]
            n112 = call-dynamic "Write.vi"("reference in"=w337, "Data"=w334, "Name"=w335, "error in (no error)"=w338) -> ("error out"=w336:errorcluster)  [unwired: 8 in, 3 out]
          }
          frame Enabled {
          }
        }
      }
      frame "Action: Update Indicators" {
      }
      frame "Action: Update Channels TBL" {
        n113 = disable-structure shown="Disabled" {
          disable-tunnel: w350 -> [w357 _]
          frame Disabled {
            n114 = Unbundle By Name(w357) -> ("Channels data"=w355)
            n115 = for {
              tunnel: T4[] [{"Name"="Уровень  масла", "SensorID"=0}, {"Name"="Уровень  масла", "SensorID"=0}, {"Name"="Температура масла", "SensorID"=0}, {"Name"="Температура масла", "SensorID"=0}, {"Name"="давление после насоса ВД", "SensorID"=0}, {"Name"="Давление в образце", "SensorID"=0}, {"Name"="Давление в камере", "SensorID"=0}, {"Name"="Давление  в  линии подачи воздуха в  блок ППВ", "SensorID"=0}, {"Name"="Давление  в  линии подачи воздуха после блока ППВ", "SensorID"=0}, {"Name"="Датчик давления в линии измерения утечек", "SensorID"=0}] ("Calibration Data") -> [w361] mode=indexing
              tunnel: w355 -> [w363]
              tunnel: [w358] -> w354 mode=indexing
              i -> [w362]
              n116 = Index Array(array=w363, index=w362) -> (element=w360)
              n117 = Unbundle By Name(w360) -> ("SensorID"=w359)
              n118 = Bundle By Name(cluster=w361, "SensorID"=w359) -> (w358:T4)
            }
            n119 = local write item#-1(w354) -> ()
          }
          frame Enabled {
          }
        }
      }
    }
  }
  n120 = call "Read SVW.vi"("GUI in"=w2) -> ("SharedVariableWrapper.lvclass"=w1:refnum<class "SharedVariableWrapper.lvclass">)  [unwired: 10 in]
  n121 = while {
    tunnel: w1 -> [w368]
    stop <- "stop" stop-if-true
    n122 = stacked-sequence {
      tunnel: w368 -> [w386 w410]
      tunnel: [w377 _] -> w366
      tunnel: [_ w394] -> w367
      frame #0 {
        n123 = control-ref of="AI 8"() -> (w380:refnum<vi>)
        n124 = control-ref of="AI 9"() -> (w379:refnum<vi>)
        n125 = call "Read.vim"("SharedVariableWrapper in"=w386, "name"="AI_DATA_ARRAY", "DataType"=T12 [] ("AI_Data_Array")) -> ("connected"=w383:bool, "data out"=w376:T12, "error out"=w382:errorcluster)  [unwired: 6 in, 4 out]
        n126 = Build Array(w380, w379) -> (w378:refnum<vi>[])
        n127 = call <vilib>:"Clear Errors.vi"("error in (no error)"=w382) -> ("error out"=w381:errorcluster)  [unwired: 5 in, 1 out]
        n128 = Index Array(array=w376, index #1=8 ("index"), index #2=9 ("index")) -> (element #1=w375:T13, element #2=w374:T13)
        n129 = Build Array(w375, w374) -> (w371:T13[])
        n130 = for {
          tunnel: w383 -> [w390]
          tunnel: w371 -> [w391]
          shift-right: [w392] -> w377
          shift-left: w381 -> [w393]
          tunnel: w378 -> [w387] mode=indexing
          i -> [w388]
          n131 = Index Array(array=w391, index=w388) -> (element=w389:T13)
          n132 = call "UpdateNumericWithScale.vi"("NumericWithScale in"=w387, "connect"=w390, "AI_Data"=w389, "error in (no error)"=w393) -> ("error out"=w392:errorcluster)  [unwired: 11 in]
        }
      }
      frame #1 {
        n133 = call "Read.vim"("SharedVariableWrapper in"=w410, "name"="DI_ARRAY", "DataType"=bool[] []) -> ("data out"=w395:bool[], "error out"=w394:errorcluster)  [unwired: 6 in, 5 out]
        n134 = Index Array(array=w395) -> (element #1=→"DI 0":bool, element #2=→"DI 1":bool, element #3=→"DI 2":bool, element #4=→"DI 3":bool, element #5=→"DI 4":bool, element #6=→"DI 5":bool, element #7=→"DI 6":bool, element #8=→"DI 7":bool, element #9=→"DI 8":bool, element #10=→"DI 9":bool, element #11=→"DI 10":bool, element #12=→"DI 11":bool)  [unwired: 12 in]
      }
    }
    n135 = Merge Errors(w367, w366) -> (w365:errorcluster)
    n136 = Wait Until Next ms Multiple(millisecond multiple=u32 100) -> ()  [unwired: 1 out]
    n137 = Unbundle By Name(w365) -> ("status"=→"Connect":bool)
  }
  n138 = flat-sequence {
    tunnel: w7 -> [w412]
    frame #0 {
      n139 = local write "stop"(TRUE ("stop")) -> ()
      "error out" <- w412
    }
  }
